vi "raw io.vi"() -> (4 "Analog I/O":T2, 6 "Relay":cluster{"Forward":bool[], "Reverse":bool[]}, 8 "PWM":cluster{u8, u8}[](array[slide])=[{128, 128}, {128, 128}, {128, 128}, {128, 128}, {128, 128}, {128, 128}, {128, 128}, {128, 128}, {128, 128}, {128, 128}] scale=1.0..255.0, 10 "GPIO State":bool[](array[boolean]), 14 "Solenoids":T1, 15 "GPIO Output Enable":bool[](array[boolean]))   [LabVIEW 2014]
uses:
  <vilib>/Rock Robotics/WPI/DriverStation/WPI_DriverStationDigitalData.ctl
  <vilib>/Rock Robotics/Network Tables/NT Read Numeric Array.vi
  <vilib>/Rock Robotics/Network Tables/NT Read Boolean Array.vi
  <vilib>/Rock Robotics/Network Tables/NT Read String.vi
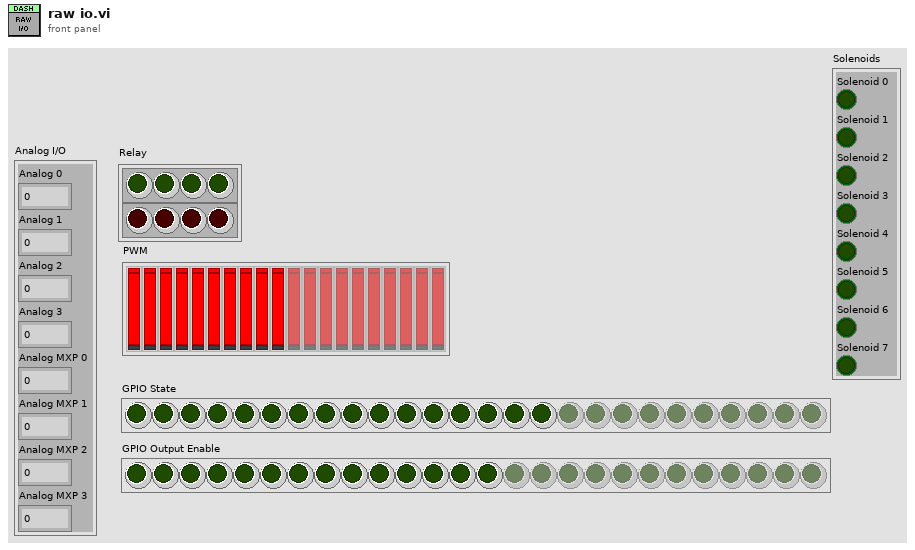
[diagram p1: front panel]
types:
  T1 = cluster{"Solenoid 0":bool, "Solenoid 1":bool, "Solenoid 2":bool, "Solenoid 3":bool, "Solenoid 4":bool, "Solenoid 5":bool, "Solenoid 6":bool, "Solenoid 7":bool}
  T2 = cluster{"Analog 0":dbl, "Analog 1":dbl, "Analog 2":dbl, "Analog 3":dbl, "Analog MXP 0":dbl, "Analog MXP 1":dbl, "Analog MXP 2":dbl, "Analog MXP 3":dbl}
  T3 = typedef "WPI_DriverStationDigitalData.ctl" = cluster{"Relay Fwd":u8, "Relay Rev":u8, "GPIO":u16, "GPIO_OE":u16, "PWM":cluster{"PWM[0]":u8, "PWM[1]":u8, "PWM[2]":u8, "PWM[3]":u8, "PWM[4]":u8, "PWM[5]":u8, "PWM[6]":u8, "PWM[7]":u8, "PWM[8]":u8, "PWM[9]":u8, "PWM[10]":u8, "PWM[11]":u8, "PWM[12]":u8, "PWM[13]":u8, "PWM[14]":u8, "PWM[15]":u8, "PWM[16]":u8, "PWM[17]":u8, "PWM[18]":u8, "PWM[19]":u8}}
  T4 = cluster{"PWM[0]":u8, "PWM[1]":u8, "PWM[2]":u8, "PWM[3]":u8, "PWM[4]":u8, "PWM[5]":u8, "PWM[6]":u8, "PWM[7]":u8, "PWM[8]":u8, "PWM[9]":u8, "PWM[10]":u8, "PWM[11]":u8, "PWM[12]":u8, "PWM[13]":u8, "PWM[14]":u8, "PWM[15]":u8, "PWM[16]":u8, "PWM[17]":u8, "PWM[18]":u8, "PWM[19]":u8}
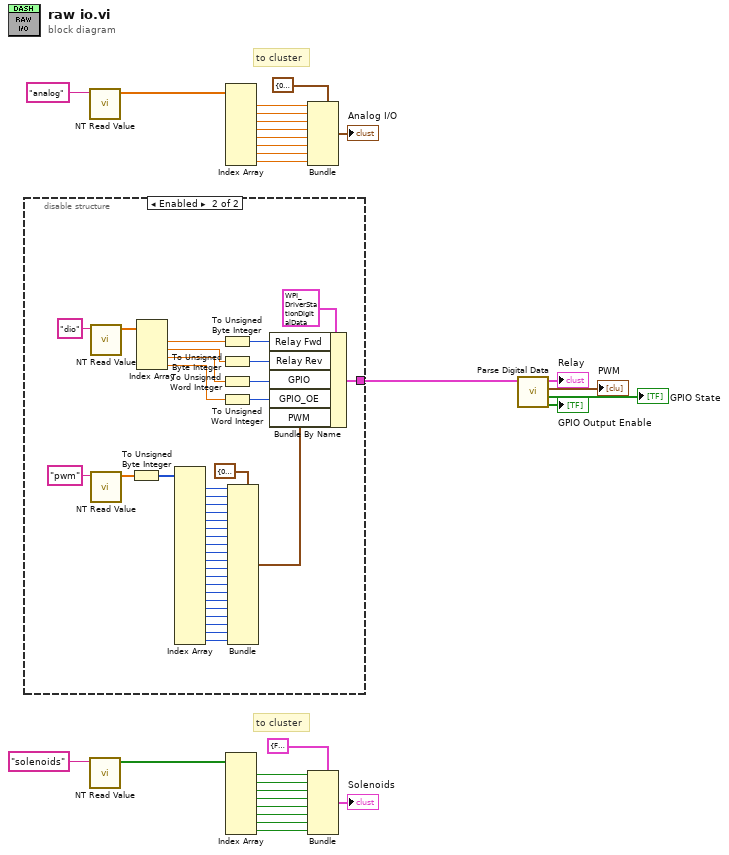
[diagram p0: block diagram]
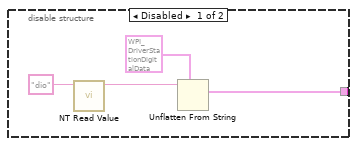
[diagram p2: hidden frame]
diagram:
  # "to cluster"
  # "to cluster"
  n1 = disable-structure shown="Enabled" {
    disable-tunnel: [w30 w67] -> w17
    frame Disabled {
      n2 = call-poly <vilib>:"NT Read Value.vi"("Name"="dio") -> ("String"=w32:string)  [unwired: 9 in, 1 out]
      n3 = Unflatten From String(type=T3 {"Relay Fwd"=0, "Relay Rev"=0, "GPIO"=0, "GPIO_OE"=0, "PWM"={"PWM[0]"=0, "PWM[1]"=0, "PWM[2]"=0, "PWM[3]"=0, "PWM[4]"=0, "PWM[5]"=0, "PWM[6]"=0, "PWM[7]"=0, "PWM[8]"=0, "PWM[9]"=0, "PWM[10]"=0, "PWM[11]"=0, "PWM[12]"=0, "PWM[13]"=0, "PWM[14]"=0, "PWM[15]"=0, "PWM[16]"=0, "PWM[17]"=0, "PWM[18]"=0, "PWM[19]"=0}} ("DigitalModule"), binary string=w32) -> (value=w30:T3)  [unwired: 3 in, 2 out]
    }
    frame Enabled {
      n4 = call-poly <vilib>:"NT Read Value.vi"("Name"="dio") -> ("Numeric Array"=w66:dbl[])  [unwired: 9 in, 1 out]
      n5 = call-poly <vilib>:"NT Read Value.vi"("Name"="pwm") -> ("Numeric Array"=w57:dbl[])  [unwired: 9 in, 1 out]
      n6 = To Unsigned Byte Integer(number=w57) -> (unsigned 8bit integer=w56:u8[])
      n7 = Index Array(array=w66) -> (element #1=w65:dbl, element #2=w62:dbl, element #3=w60:dbl, element #4=w58:dbl)  [unwired: 4 in]
      n8 = Index Array(array=w56) -> (element #1=w54:u8, element #2=w55:u8, element #3=w36:u8, element #4=w37:u8, element #5=w38:u8, element #6=w39:u8, element #7=w40:u8, element #8=w41:u8, element #9=w42:u8, element #10=w43:u8, element #11=w44:u8, element #12=w45:u8, element #13=w46:u8, element #14=w47:u8, element #15=w48:u8, element #16=w49:u8, element #17=w50:u8, element #18=w51:u8, element #19=w52:u8, element #20=w53:u8)  [unwired: 20 in]
      n9 = To Unsigned Byte Integer(number=w65) -> (unsigned 8bit integer=w64:u8)
      n10 = To Unsigned Byte Integer(number=w62) -> (unsigned 8bit integer=w63:u8)
      n11 = To Unsigned Word Integer(number=w60) -> (unsigned 16bit integer=w61:u16)
      n12 = To Unsigned Word Integer(number=w58) -> (unsigned 16bit integer=w59:u16)
      n13 = Bundle(cluster=T4 {"PWM[0]"=0, "PWM[1]"=0, "PWM[2]"=0, "PWM[3]"=0, "PWM[4]"=0, "PWM[5]"=0, "PWM[6]"=0, "PWM[7]"=0, "PWM[8]"=0, "PWM[9]"=0, "PWM[10]"=0, "PWM[11]"=0, "PWM[12]"=0, "PWM[13]"=0, "PWM[14]"=0, "PWM[15]"=0, "PWM[16]"=0, "PWM[17]"=0, "PWM[18]"=0, "PWM[19]"=0} ("PWM"), "PWM[0]"=w54, "PWM[1]"=w55, "PWM[2]"=w36, "PWM[3]"=w37, "PWM[4]"=w38, "PWM[5]"=w39, "PWM[6]"=w40, "PWM[7]"=w41, "PWM[8]"=w42, "PWM[9]"=w43, "PWM[10]"=w44, "PWM[11]"=w45, "PWM[12]"=w46, "PWM[13]"=w47, "PWM[14]"=w48, "PWM[15]"=w49, "PWM[16]"=w50, "PWM[17]"=w51, "PWM[18]"=w52, "PWM[19]"=w53) -> (w35:T4)
      n14 = Bundle By Name(cluster=T3 {"Relay Fwd"=0, "Relay Rev"=0, "GPIO"=0, "GPIO_OE"=0, "PWM"={"PWM[0]"=0, "PWM[1]"=0, "PWM[2]"=0, "PWM[3]"=0, "PWM[4]"=0, "PWM[5]"=0, "PWM[6]"=0, "PWM[7]"=0, "PWM[8]"=0, "PWM[9]"=0, "PWM[10]"=0, "PWM[11]"=0, "PWM[12]"=0, "PWM[13]"=0, "PWM[14]"=0, "PWM[15]"=0, "PWM[16]"=0, "PWM[17]"=0, "PWM[18]"=0, "PWM[19]"=0}} ("DigitalModule"), "Relay Fwd"=w64, "Relay Rev"=w63, "GPIO"=w61, "GPIO_OE"=w59, "PWM"=w35) -> (w67:T3)
    }
  }
  n15 = call-poly <vilib>:"NT Read Value.vi"("Name"="analog") -> ("Numeric Array"=w28:dbl[])  [unwired: 9 in, 1 out]
  n16 = call-poly <vilib>:"NT Read Value.vi"("Name"="solenoids") -> ("Boolean Array"=w11:bool[])  [unwired: 9 in, 1 out]
  n17 = Index Array(array=w28) -> (element #1=w26:dbl, element #2=w25:dbl, element #3=w24:dbl, element #4=w23:dbl, element #5=w22:dbl, element #6=w21:dbl, element #7=w20:dbl, element #8=w19:dbl)  [unwired: 8 in]
  n18 = Index Array(array=w11) -> (element #1=w9:bool, element #2=w8:bool, element #3=w7:bool, element #4=w6:bool, element #5=w5:bool, element #6=w4:bool, element #7=w3:bool, element #8=w2:bool)  [unwired: 8 in]
  n19 = Bundle(cluster=T2 {"Analog 0"=0.0, "Analog 1"=0.0, "Analog 2"=0.0, "Analog 3"=0.0, "Analog MXP 0"=0.0, "Analog MXP 1"=0.0, "Analog MXP 2"=0.0, "Analog MXP 3"=0.0}, "Analog 0"=w26, "Analog 1"=w25, "Analog 2"=w24, "Analog 3"=w23, "Analog MXP 0"=w22, "Analog MXP 1"=w21, "Analog MXP 2"=w20, "Analog MXP 3"=w19) -> (→"Analog I/O":T2)
  n20 = Bundle(cluster=T1 {"Solenoid 0"=FALSE, "Solenoid 1"=FALSE, "Solenoid 2"=FALSE, "Solenoid 3"=FALSE, "Solenoid 4"=FALSE, "Solenoid 5"=FALSE, "Solenoid 6"=FALSE, "Solenoid 7"=FALSE}, "Solenoid 0"=w9, "Solenoid 1"=w8, "Solenoid 2"=w7, "Solenoid 3"=w6, "Solenoid 4"=w5, "Solenoid 5"=w4, "Solenoid 6"=w3, "Solenoid 7"=w2) -> (→"Solenoids":T1)
  n21 = call "Parse Digital Data.vi"("DigitalModule"=w17) -> ("GPIO Output Enable"=→"GPIO Output Enable":bool[], "GPIO State"=→"GPIO State":bool[], "PWM"=→"PWM":cluster{u8, u8}[], "Relay"=→"Relay":cluster{"Forward":bool[], "Reverse":bool[]})  [unwired: 7 in]
